vi "SPI_Get_Device Details.vi"(0 "DeviceIndex":u32) -> (1 "FTC_Status":u32, 2 "DeviceName":string, 3 "LocID":u32 format="%x")   [LabVIEW 2010]
uses:
  WINNT/system32/FTCSPI.dll
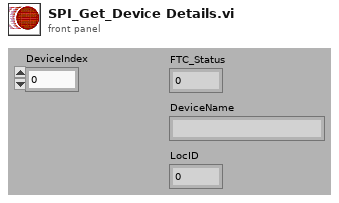
[diagram p1: front panel]
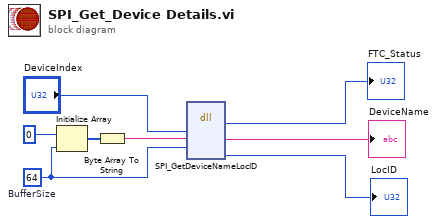
[diagram p0: block diagram]
diagram:
  w1 = u32 64  # BufferSize
  n1 = Initialize Array(u8 0 ("element"), w1) -> (w3:u8[])
  n2 = Byte Array To String(unsigned byte array=w3) -> (string=w2:string)
  n3 = dll-call lib="C:/Users/WINNT/system32/FTCSPI.dll" fn="SPI_GetDeviceNameLocID"("DeviceIndex"="DeviceIndex", "DeviceNameBuffer"=w2, "BufferSize"=w1) -> ("FTC_Status"=→"FTC_Status":u32, "DeviceNameBuffer"=→"DeviceName":string, "LocID"=→"LocID":u32)  [unwired: 6 in, 2 out]
